vi "例3.4 字符串的分解.vi"() -> ()   [LabVIEW 2012]
panel:
  out "数值":dbl
  in  "偏移量(0) 2":i32=9
  out "子字符串":string
  in  "长度（剩余）":i32=2
  in  "偏移量(0)":i32=6
  in  "输入字符串":string="VOLTS DC +1.345E+02"
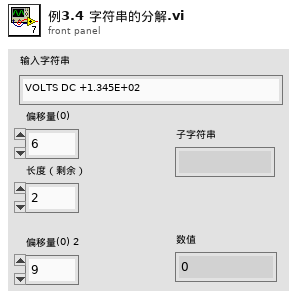
[diagram p1: front panel]
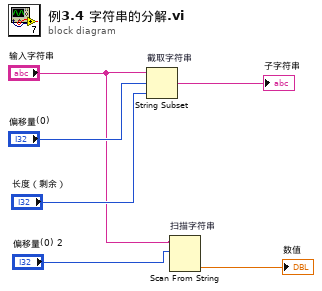
[diagram p0: block diagram]
diagram:
  n1 = String Subset "截取字符串"(string="输入字符串", offset (0)="偏移量(0)", length (rest)="长度（剩余）") -> (substring=→"子字符串":string)
  n2 = Scan From String "扫描字符串"(input string="输入字符串", initial scan location="偏移量(0) 2") -> (output 1=→"数值":dbl)  [unwired: 3 in, 3 out]
